vi "soundsubVI.vi"(8 "error in (no error)":errorcluster, 10 "Sound File 2":path, 11 "Sound File 1":path) -> (0 "error out":errorcluster, 1 "Sound graph of Combined":waveform(dbl)[](graph), 2 "Sound graph of 2":waveform(dbl)[](graph), 3 "Sound graph of 1":waveform(dbl)[](graph))   [LabVIEW 2014]
uses:
  <vilib>/sound2/lvsound2.llb/Sound File Read Open.vi
  <vilib>/sound2/lvsound2.llb/Sound File Read (DBL).vi
  <vilib>/sound2/lvsound2.llb/Sound Output Write (DBL).vi
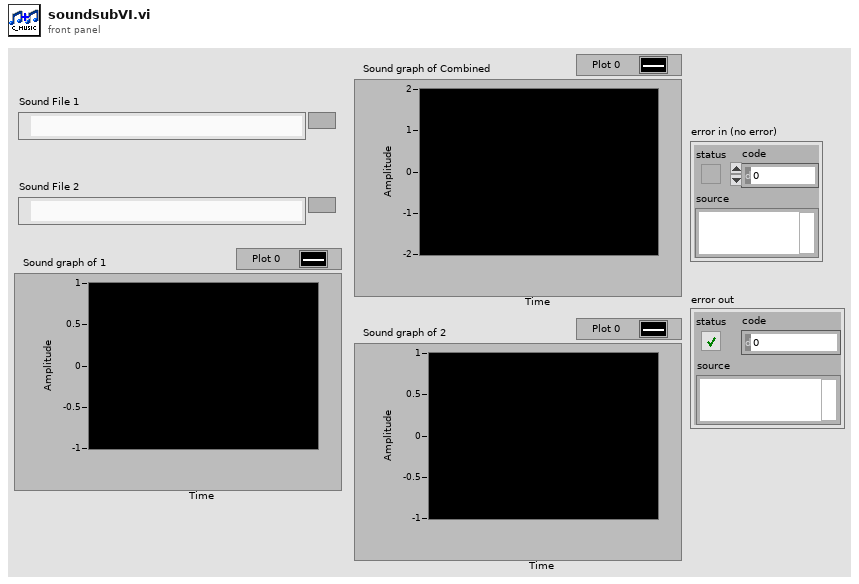
[diagram p1: front panel]
types:
  T1 = typedef "Sound File Refnum.ctl" = refnum<file>
  T2 = typedef "Sound Output Task ID.ctl" = u32
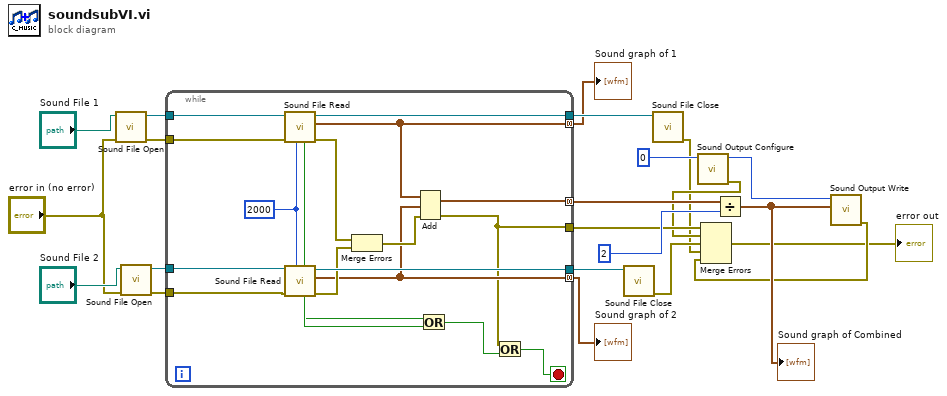
[diagram p0: block diagram]
diagram:
  n1 = call-poly <vilib>:"Sound File Open.vi"("error in (no error)"="error in (no error)", "path"="Sound File 1") -> ("error out"=w18:errorcluster, "sound file refnum"=w17:T1)  [unwired: 8 in]
  n2 = call-poly <vilib>:"Sound File Open.vi"("error in (no error)"="error in (no error)", "path"="Sound File 2") -> ("error out"=w21:errorcluster, "sound file refnum"=w20:T1)  [unwired: 8 in]
  n3 = while {
    tunnel: w21 -> [w39]
    tunnel: w20 -> [w38]
    tunnel: w18 -> [w37]
    tunnel: w17 -> [w36]
    tunnel: [w26] -> w11 mode=concatenating
    tunnel: [w25] -> w12 mode=concatenating
    tunnel: [w35] -> w14
    tunnel: [w34] -> w13
    tunnel: [w24] -> w10 mode=concatenating
    tunnel: [w23] -> w7
    stop <- w29 stop-if-true
    w40 = 2000
    n4 = call-poly <vilib>:"Sound File Read.vi"("number of samples/ch (-1: all)"=w40, "error in (no error)"=w37, "sound file refnum"=w36) -> ("error out"=w32:errorcluster, "data"=w25:waveform(dbl)[], "sound file refnum out"=w35:T1, "end of file?"=w30:bool)  [unwired: 4 in, 1 out]
    n5 = call-poly <vilib>:"Sound File Read.vi"("number of samples/ch (-1: all)"=w40, "error in (no error)"=w39, "sound file refnum"=w38) -> ("error out"=w33:errorcluster, "data"=w26:waveform(dbl)[], "sound file refnum out"=w34:T1, "end of file?"=w31:bool)  [unwired: 4 in, 1 out]
    n6 = Merge Errors(w32, w33) -> (w28:errorcluster)
    n7 = Add(1:w26, 2:w25, 4:w28) -> (0:w24:waveform(dbl)[], 3:w23:errorcluster)
    n8 = Or(x=w30, y=w31) -> (x .or. y?=w27:bool)
    n9 = Or(x=w23, y=w27) -> (x .or. y?=w29:bool)
  }
  "Sound graph of 1" <- w12
  "Sound graph of 2" <- w11
  n10 = call <vilib>:"Sound File Close.vi"("sound file refnum"=w13) -> ("error out"=w5:errorcluster)  [unwired: 10 in]
  n11 = call <vilib>:"Sound File Close.vi"("sound file refnum"=w14) -> ("error out"=w4:errorcluster)  [unwired: 10 in]
  n12 = call <vilib>:"Sound Output Configure.vi"("device ID"=0) -> ("error out"=w6:errorcluster, "task ID"=w15:T2)  [unwired: 9 in]
  n13 = Divide(x=w10, y=2) -> (x/y=w8:waveform(dbl)[])
  "Sound graph of Combined" <- w8
  n14 = call-poly <vilib>:"Sound Output Write.vi"("data"=w8, "task ID"=w15) -> ("error out"=w3:errorcluster)  [unwired: 8 in, 1 out]
  n15 = Merge Errors(w7, w6, w5, w4, w3) -> (→"error out":errorcluster)
